vi "FFT1D_LabVIEW.vi"(7 "Iteration":i32, 11 "Samples":i32) -> (3 "Results(s)":dbl format="%.8f")   [LabVIEW 2020]
uses:
  ec656ee5-c5d1-4756-bc0c-4372cb75bedf.vi
  <vilib>/Analysis/2dsp.llb/Complex FFT.vi
  88f9a4a6-1eb4-4671-a21a-3a41d51d2300.vi
  <vilib>/Utility/High Resolution Relative Seconds.vi
  <vilib>/Analysis/NI_AALBase.lvlib
  <vilib>/Analysis/NI_AALPro.lvlib
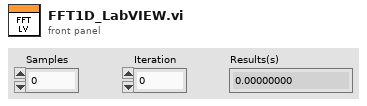
[diagram p1: front panel]
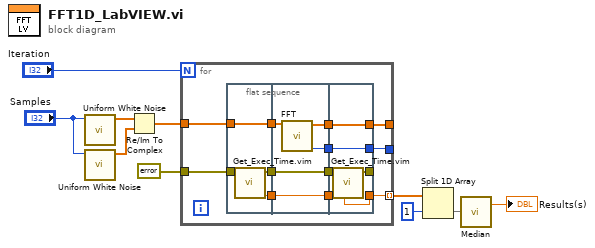
[diagram p0: block diagram]
diagram:
  n1 = call <vilib>:"Uniform White Noise.vi"("samples"="Samples") -> ("uniform white noise"=w4:dbl[])  [unwired: 9 in, 1 out]
  n2 = call <vilib>:"Uniform White Noise.vi"("samples"="Samples") -> ("uniform white noise"=w5:dbl[])  [unwired: 9 in, 1 out]
  n3 = Re/Im To Complex(1:w5, 2:w4) -> (0:w7:cdb[])
  n4 = for {
    N: "Iteration" -> [_]
    tunnel: w7 -> [w21]
    tunnel: errorcluster {"status"=FALSE, "code"=0, "source"=""} ("error out") -> [w19]
    tunnel: [w22] -> _
    tunnel: [w20] -> _
    tunnel: [w11] -> w9 mode=indexing
    n5 = flat-sequence {
      tunnel: w19 -> [w25]
      tunnel: w21 -> [w26]
      tunnel: [w26] -> w18
      tunnel: [w24] -> w17
      tunnel: [w23] -> w12
      tunnel: w18 -> [w30]
      tunnel: w17 -> [w28]
      tunnel: [w31] -> w16
      tunnel: [w29] -> w15
      tunnel: [w28] -> w14
      tunnel: [w27] -> w13
      tunnel: w12 -> [w27]
      tunnel: [w34] -> _
      tunnel: [w36] -> w20
      tunnel: [w37] -> w22
      tunnel: w16 -> [w37]
      tunnel: w15 -> [w36]
      tunnel: w14 -> [w35]
      tunnel: w13 -> [w33]
      tunnel: [w32] -> w11
      frame #0 {
        n6 = call "Get_Exec_Time.vim"("error in (no error)"=w25) -> ("T(n)"=w23:dbl, "error out"=w24:errorcluster)  [unwired: 6 in, 1 out]
      }
      frame #1 {
        n7 = call-poly <vilib>:"FFT.vi"("X"=w30) -> ("error"=w31:i32, "FFT {X}"=w29:cdb[])  [unwired: 9 in]
      }
      frame #2 {
        n8 = call "Get_Exec_Time.vim"("T(n-1)"=w33, "error in (no error)"=w35) -> ("error out"=w34:errorcluster, "dT"=w32:dbl)  [unwired: 5 in, 1 out]
      }
    }
  }
  n9 = Split 1D Array(array=w9, index=1) -> (second subarray=w1:dbl[])  [unwired: 1 out]
  n10 = call <vilib>:"Median.vi"("X"=w1) -> ("median"=→"Results(s)":dbl)  [unwired: 1 out]
